vi "BLED1112-Rx Packet parser (EVENT-Disconnected).vi"(5 "message package":u8[](array[numeric])=[128, 16, 3, 0, 0, 9, 198, 109, 145, 234, 23, 0, 0, 6, 0, 100, 0, 0, 0, 255] format="%02x") -> (0 "message out":u8[](array[numeric])=[128, 16, 3, 0, 0, 9, 198, 109, 145, 234, 23, 0, 0, 6, 0, 100, 0, 0, 0, 255] format="%02x", 1 "Packet OK":bool, 2 "Data Structure":T1={"Message Type (Response)"=128, "Payload length"=16, "Command Class (Connection)"=3, "Message ID"=0, "connection"=0, "reason"=9} {"reason" format="%04x"; "Message ID" format="%02x"; "Message Type (Response)" format="%02x" items=["Command / Response"=0, "Event"=128]; "Command Class (Connection)" format="%02x" items=["System", "Persistent Store", "Attribute database", "Connection", "Attribute client", "Security Manager", "Generic Access Profile", "Hardware"]})   [LabVIEW 2015]
uses:
  Lib_Bled112 toolkit/type_def/message_type.ctl
  Lib_Bled112 toolkit/type_def/message_class.ctl
panel:
  # "Rx Packet parser (EVENT-Disconnected)"
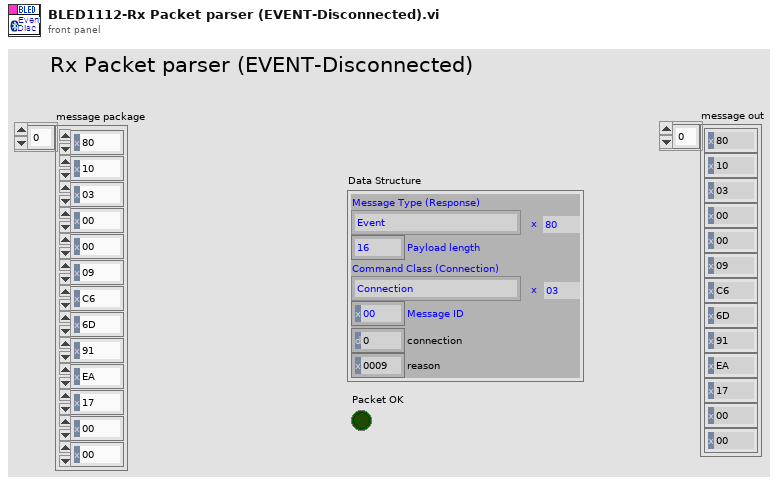
[diagram p1: front panel]
types:
  T1 = typedef "컨트롤-BLED Rx (EVENT-Disconnected).ctl" = cluster{"Message Type (Response)":T2, "Payload length":u8, "Command Class (Connection)":T3, "Message ID":u8, "connection":u8, "reason":u16}
  T2 = typedef "message_type.ctl" = u8
  T3 = typedef "message_class.ctl" = u8
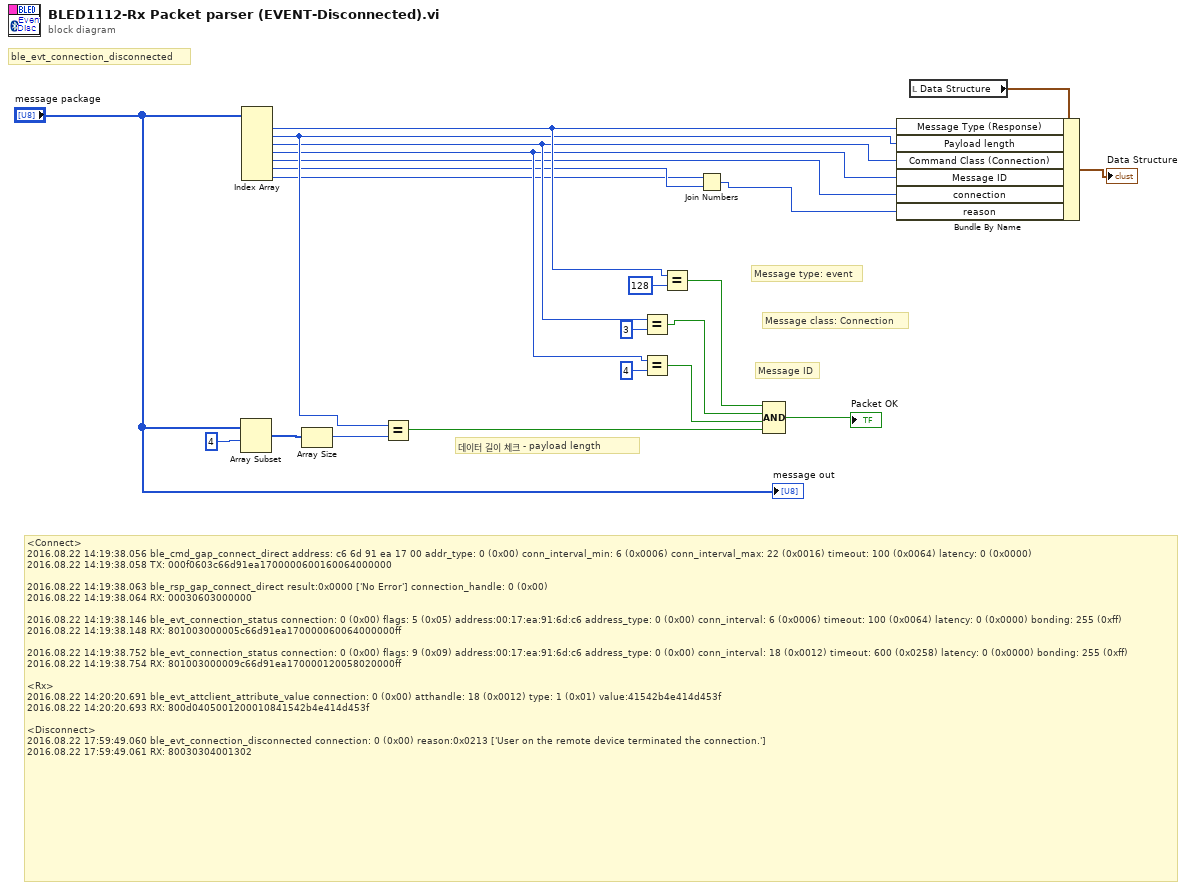
[diagram p0: block diagram]
diagram:
  # "Message type: event"
  # "ble_evt_connection_disconnected"
  # "Message ID"
  # "Message class: Connection"
  # "데이터 길이 체크 - payload length"
  # "<Connect>\n2016.08.22 14:19:38.056 ble_cmd_gap_connect_direct address: c6 6d 91 ea 17 00 addr_type: 0 (0x00) conn_interval_min: 6 (0x0006) conn_interval_max: 22 (0x0016) timeout: 100 (0x0064) latency: 0 (0x0000)\n2016.08.22 14:19:38.058 TX: 000f0603c66d91ea1700000600160064000000\n\n2016.08.22 14:19:38.063 ble_rsp_gap_connect_direct result:0x0000 ['No Error'] connection_handle: 0 (0x00)\n2016.08.22 14:19:38.064 RX: 00030603000000\n\n2016.08.22 14:19:38.146 ble_evt_connection_status connection: 0 (0x00) flags: 5 (0x05) address:00:17:ea:91:6d:c6 address_type: 0 (0x00) conn_interval: 6 (0x0006) timeout: 100 (0x0064) latency: 0 (0x0000) bonding: 255 (0xff)\n2016.08.22 14:19:38.148 RX: 801003000005c66d91ea170000060064000000ff\n\n2016.08.22 14:19:38.752 ble_evt_connection_status connection: 0 (0x00) flags: 9 (0x09) address:00:17:ea:91:6d:c6 address_type: 0 (0x00) conn_interval: 18 (0x0012) timeout: 600 (0x0258) latency: 0 (0x0000) bonding: 255 (0xff)\n2016.08.22 14:19:38.754 RX: 801003000009c66d91ea170000120058020000ff\n\n<Rx>\n2016.08.22 14:20:20.691 ble_evt_attclient_attribute_value connection: 0 (0x00) atthandle: 18 (0x0012) type: 1 (0x01) value:41542b4e414d453f\n2016.08.22 14:20:20.693 RX: 800d0405001200010841542b4e414d453f\n\n<Disconnect>\n2016.08.22 17:59:49.060 ble_evt_connection_disconnected connection: 0 (0x00) reason:0x0213 ['User on the remote device terminated the connection.']\n2016.08.22 17:59:49.061 RX: 80030304001302"
  n1 = Array Subset(array="message package", index=4 ("인덱스")) -> (w19:u8[])  [unwired: 1 in]
  n2 = Index Array(array="message package") -> (element #1=w8:u8, element #2=w7:u8, element #3=w6:u8, element #4=w5:u8, element #5=w4:u8, element #6=w3:u8, element #7=w2:u8)  [unwired: 7 in]
  n3 = Array Size(array=w19) -> (size(s)=w18:i32)
  n4 = Equal?(x=w7, y=w18) -> (x = y?=w21:bool)
  n5 = Equal?(x=w6, y=3 ("인덱스")) -> (x = y?=w13:bool)
  n6 = Equal?(x=w5, y=4 ("인덱스")) -> (x = y?=w14:bool)
  n7 = Equal?(x=w8, y=128 ("인덱스")) -> (x = y?=w11:bool)
  n8 = Join Numbers(hi=w2, lo=w3) -> ((hi.lo)=w1:u16)
  n9 = Compound Arithmetic op=AND ("복합 연산")(w11, w13, w14, w21) -> (→"Packet OK":bool)
  n10 = local read "Data Structure"() -> (w10:T1)
  n11 = Bundle By Name(cluster=w10, "Message Type (Response)"=w8, "Payload length"=w7, "Command Class (Connection)"=w6, "Message ID"=w5, "connection"=w4, "reason"=w1) -> (→"Data Structure":T1)
  "message out" <- "message package"
